vi "GNC-1.vi"(11 "数组":u8[](array[numeric])) -> (1 "传感器信号":cluster{"陀螺温度":i32, "加速度计温度":i32}, 2 "加速度":cluster{"X轴加速度":i32, "Y轴加速度":i32, "Z轴加速度":i32}, 3 "角速度":cluster{"X轴角速度":i32, "Y轴角速度":i32, "Z轴角速度":i32}, 4 "数据有效性标志":cluster{" 加速度计":bool, "陀螺数据":bool})   [LabVIEW 2012]
uses:
  index-i32.vi
  XX-I32.vi
  index-i8.vi
panel:
  out "测量数据有效性标记":string
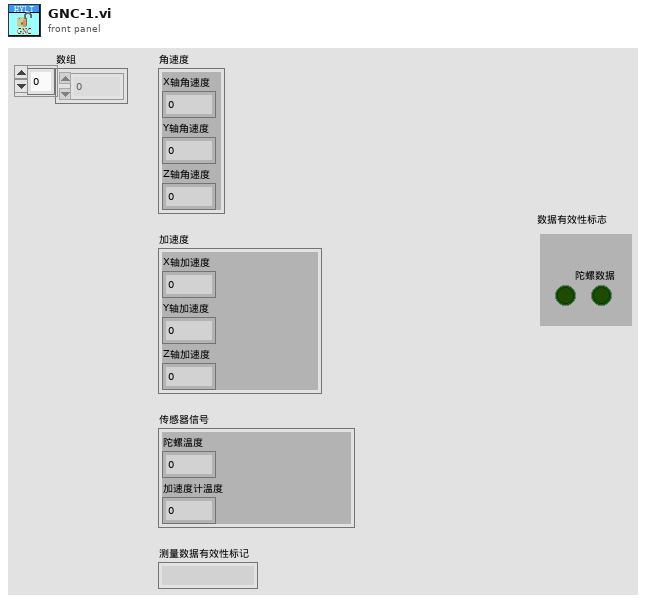
[diagram p1: front panel]
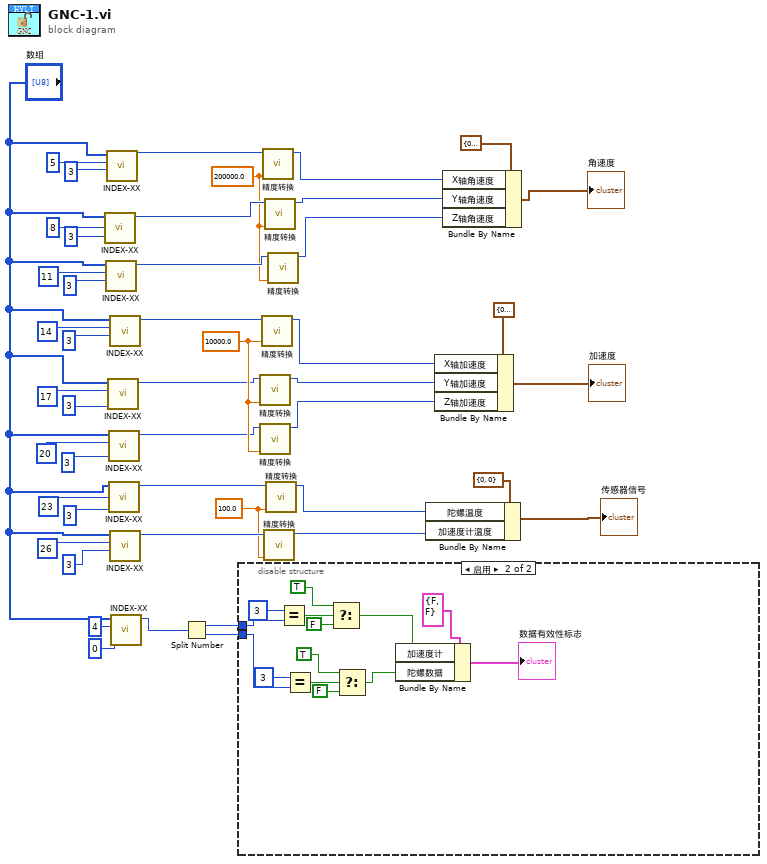
[diagram p0: block diagram]
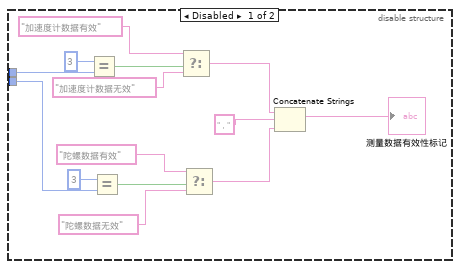
[diagram p2: hidden frame]
diagram:
  w39 = 100.0 ("单位")
  w36 = 10000.0 ("单位")
  w25 = 200000.0 ("单位")
  n1 = call-poly "INDEX-XX.vi"("长度"=3, "索引"=8, "数组"="数组") -> ("数值输出"=w26:i32)  [unwired: 8 in]
  n2 = call-poly "INDEX-XX.vi"("长度"=3, "索引"=11, "数组"="数组") -> ("数值输出"=w27:i32)  [unwired: 8 in]
  n3 = call-poly "INDEX-XX.vi"("长度"=3, "索引"=5, "数组"="数组") -> ("数值输出"=w23:i32)  [unwired: 8 in]
  n4 = call-poly "INDEX-XX.vi"("长度"=3, "索引"=17, "数组"="数组") -> ("数值输出"=w34:i32)  [unwired: 8 in]
  n5 = call-poly "INDEX-XX.vi"("长度"=3, "索引"=20, "数组"="数组") -> ("数值输出"=w35:i32)  [unwired: 8 in]
  n6 = call-poly "INDEX-XX.vi"("长度"=3, "索引"=23, "数组"="数组") -> ("数值输出"=w37:i32)  [unwired: 8 in]
  n7 = call-poly "INDEX-XX.vi"("长度"=3, "索引"=14, "数组"="数组") -> ("数值输出"=w30:i32)  [unwired: 8 in]
  n8 = call-poly "INDEX-XX.vi"("长度"=3, "索引"=26, "数组"="数组") -> ("数值输出"=w40:i32)  [unwired: 8 in]
  n9 = call-poly "INDEX-XX.vi"("长度"=0, "索引"=4, "数组"="数组") -> ("数值输出"=w45:i8)  [unwired: 8 in]
  n10 = Split Number(x=w45) -> (hi(x)=w46:u8, lo(x)=w47:u8)
  n11 = disable-structure shown="启用" {
    disable-tunnel: w47 -> [w53 w66]
    disable-tunnel: w46 -> [w48 w75]
    frame Disabled {
      n12 = Equal?(x=u16 3, y=w48) -> (x = y?=w50:bool)
      n13 = Equal?(x=u16 3, y=w53) -> (x = y?=w51:bool)
      n14 = Select(t="加速度计数据有效", s=w50, f="加速度计数据无效") -> (s? t:f=w58:string)
      n15 = Select(t="陀螺数据有效", s=w51, f="陀螺数据无效") -> (s? t:f=w60:string)
      n16 = Concatenate Strings(w58, "，", w60) -> (→"测量数据有效性标记":string)
    }
    frame Enabled {
      n17 = Equal?(x=u8 3, y=w75) -> (x = y?=w73:bool)
      n18 = Equal?(x=u8 3, y=w66) -> (x = y?=w68:bool)
      n19 = Select(t=TRUE, s=w73, f=FALSE) -> (s? t:f=w65:bool)
      n20 = Select(t=TRUE, s=w68, f=FALSE) -> (s? t:f=w64:bool)
      n21 = Bundle By Name(cluster=cluster{" 加速度计":bool, "陀螺数据":bool} {" 加速度计"=FALSE, "陀螺数据"=FALSE} ("数据有效性标志"), "加速度计"=w65, "陀螺数据"=w64) -> (→"数据有效性标志":cluster{" 加速度计":bool, "陀螺数据":bool})
    }
  }
  n22 = call-poly "精度转换.vi"("单位"=w36, "数值输入"=w34) -> ("输出"=w32:i32)  [unwired: 9 in]
  n23 = call-poly "精度转换.vi"("单位"=w36, "数值输入"=w35) -> ("输出"=w33:i32)  [unwired: 9 in]
  n24 = call-poly "精度转换.vi"("单位"=w36, "数值输入"=w30) -> ("输出"=w31:i32)  [unwired: 9 in]
  n25 = call-poly "精度转换.vi"("单位"=w25, "数值输入"=w23) -> ("输出"=w24:i32)  [unwired: 9 in]
  n26 = call-poly "精度转换.vi"("单位"=w39, "数值输入"=w40) -> ("输出"=w41:i32)  [unwired: 9 in]
  n27 = call-poly "精度转换.vi"("单位"=w25, "数值输入"=w26) -> ("输出"=w28:i32)  [unwired: 9 in]
  n28 = call-poly "精度转换.vi"("单位"=w39, "数值输入"=w37) -> ("输出"=w38:i32)  [unwired: 9 in]
  n29 = call-poly "精度转换.vi"("单位"=w25, "数值输入"=w27) -> ("输出"=w29:i32)  [unwired: 9 in]
  n30 = Bundle By Name(cluster=cluster{"陀螺温度":i32, "加速度计温度":i32} {"陀螺温度"=0, "加速度计温度"=0} ("传感器信号"), "陀螺温度"=w38, "加速度计温度"=w41) -> (→"传感器信号":cluster{"陀螺温度":i32, "加速度计温度":i32})
  n31 = Bundle By Name(cluster=cluster{"X轴加速度":i32, "Y轴加速度":i32, "Z轴加速度":i32} {"X轴加速度"=0, "Y轴加速度"=0, "Z轴加速度"=0} ("加速度"), "X轴加速度"=w31, "Y轴加速度"=w32, "Z轴加速度"=w33) -> (→"加速度":cluster{"X轴加速度":i32, "Y轴加速度":i32, "Z轴加速度":i32})
  n32 = Bundle By Name(cluster=cluster{"X轴角速度":i32, "Y轴角速度":i32, "Z轴角速度":i32} {"X轴角速度"=0, "Y轴角速度"=0, "Z轴角速度"=0} ("角速度"), "X轴角速度"=w24, "Y轴角速度"=w28, "Z轴角速度"=w29) -> (→"角速度":cluster{"X轴角速度":i32, "Y轴角速度":i32, "Z轴角速度":i32})
